vi "Command Handler.vi"(8 "error in (no error)":errorcluster, 10 "command":T1, 11 "Thread in":refnum<class "Thread.lvclass">) -> (0 "error out":errorcluster, 1 "shutdown?":bool, 3 "Thread out":refnum<class "Thread.lvclass">)   [LabVIEW 2017, in "DSF Core.lvlib" / "Thread.lvclass"]
uses:
  Thread.lvclass
  Thread State.ctl
  Thread Command.ctl
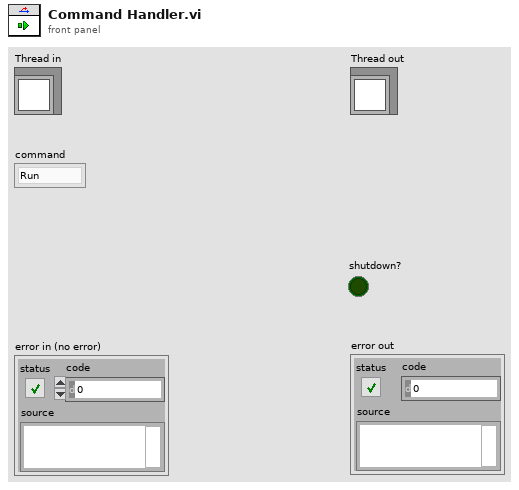
[diagram p1: front panel]
types:
  T1 = typedef "DSF Core.lvlib/Thread.lvclass/Thread Command.ctl" = enum8{"Run", "Shutdown"}
  T2 = typedef "DSF Core.lvlib/Thread.lvclass/Thread State.ctl" = enum8{"Idle", "Running", "Error", "Shut Down"}
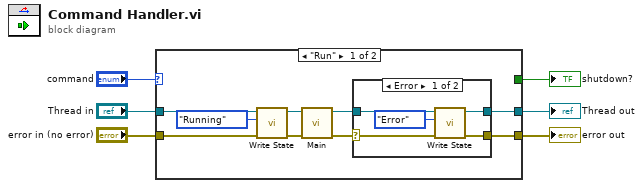
[diagram p0: block diagram]
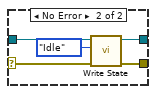
[diagram p2: hidden frame]
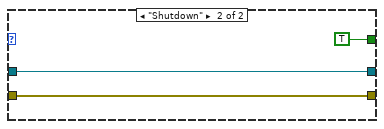
[diagram p3: hidden frame]
diagram:
  n1 = case shown="\"Run\"" "command" {
    tunnel: "error in (no error)" -> [w14 w26]
    tunnel: [w7 w26] -> w2
    tunnel: [w8 w27] -> w3
    tunnel: "Thread in" -> [w15 w27]
    tunnel: [_ TRUE] -> w1
    frame "Run" {
      n2 = call "Write State.vi"("error in (no error)"=w14, "state"=Thread_State."Running", "Thread in"=w15) -> ("error out"=w12:errorcluster, "Thread out"=w13:refnum<class "Thread.lvclass">)  [unwired: 7 in]
      n3 = call-dynamic "Main.vi"("error in (no error)"=w12, "Thread in"=w13) -> ("error out"=w10:errorcluster, "Thread out"=w9:refnum<class "Thread.lvclass">)  [unwired: 8 in]
      n4 = case shown="Error" w10 {
        selector: w10 -> [w18 w23]
        tunnel: w9 -> [w19 w24]
        tunnel: [w17 w22] -> w8
        tunnel: [w16 w21] -> w7
        frame Error {
          n5 = call "Write State.vi"("error in (no error)"=w18, "state"=Thread_State."Error", "Thread in"=w19) -> ("error out"=w16:errorcluster, "Thread out"=w17:refnum<class "Thread.lvclass">)  [unwired: 7 in]
        }
        frame No Error {
          n6 = call "Write State.vi"("error in (no error)"=w23, "state"=Thread_State."Idle", "Thread in"=w24) -> ("error out"=w21:errorcluster, "Thread out"=w22:refnum<class "Thread.lvclass">)  [unwired: 7 in]
        }
      }
    }
    frame "Shutdown" {
    }
  }
  "Thread out" <- w3
  "error out" <- w2
  "shutdown?" <- w1
